vi "Basic Demo Launcher.vi"   [LabVIEW 2017, in "2. Basic Panel Actors.lvlib"]
doc: "Launches the Panel Actor Example.\n----\nCopyright: MGI 2016\nAuthor: Derek Trepanier"
uses:
  2. Basic Panel Actors.lvlib
  Basic Demo/Basic Demo.lvclass
  D:/software/LabView_PanelManager/panel-actors/Source/Panel Actor/Panel Actor.lvclass
  panel-manager/Source/Window Position/Reference Position/Ref Display/Ref Display.lvclass
  D:/software/LabView_PanelManager/panel-manager/Source/Window Position/Window Position.lvclass
  panel-manager/Source/Window Position/Reference Position/Ref Display/Ref Display.vi
  panel-actors/Source/Launch Root Panel Window.vi
  panel-actors/Source/MGI-Panel Actor.lvlib
  panel-manager/Source/MGI-Panel Manager.lvlib
  D:/software/LabView_PanelManager/panel-manager/Source/Window Position/Reference Position/Reference Position.lvclass
  C:/Program Files (x86)/National Instruments/LabVIEW 2017/vi.lib/ActorFramework/Actor/Actor.lvclass
panel:
  # "Run this VI to launch the Panel Actor Example"
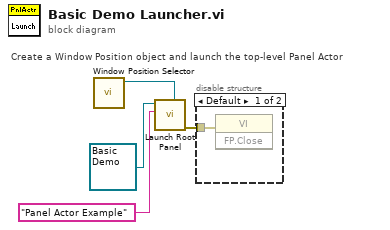
[diagram p0: block diagram]
diagram:
  # "Create a Window Position object and launch the top-level Panel Actor"
  n1 = call-poly "Window Position Selector.vi"() -> ("Ref Display out"=w1:refnum<class "Ref Display.lvclass">)  [unwired: 10 in, 1 out]
  n2 = call-poly "Launch Root Panel.vi"("Window Position (Maximize First Call)"=w1, "Title"="Panel Actor Example", "Panel Actor in"=refnum<class "Basic Demo.lvclass"> refnum ("Basic Panel Actors.lvlib:Top Level.lvclass")) -> ("Error Out"=w2:errorcluster)  [unwired: 7 in, 1 out]
  n3 = disable-structure shown="Default" {
    disable-tunnel: w2 -> [w5 _]
    frame condition #0 {
      n4 = invoke class="VI" method="FP.Close"(error in=w5) -> ()  [unwired: 2 in, 3 out]
    }
    frame condition #1 (active) {
    }
  }
